vi "acquisition test fixed exposure 5.vi"() -> ()   [LabVIEW 2023]
uses:
  <vilib>/vision/driver/IMAQdx.llb/IMAQdx Attribute Type.ctl
  <vilib>/userDefined/High Color/IMAQdx.ctl
  <vilib>/vision/driver/IMAQdx.llb/IMAQdx Acquisition Mode.ctl
  <vilib>/vision/Avi.llb/IMAQ AVI2 Refnum.ctl
  <vilib>/vision/Image Controls.llb/IMAQ Image.ctl
  <vilib>/vision/driver/IMAQdx.llb/IMAQdx Buffer Number Mode.ctl
  <extravilib>/ChannelInstances/Tag-bool/Read With Abort.vi
  <vilib>/Utility/High Resolution Relative Seconds.vi
  <extravilib>/ChannelInstances/Tag-bool/Write With Abort.vi
  <extravilib>/ChannelInstances/Tag-bool/Instantiate.vi
  <extravilib>/ChannelInstances/Tag-bool/EndpointRead.vi
  <vilib>/vision/EDVR.llb/IMAQ ImageToEDVR.vi
  <vilib>/vision/EDVR.llb/IMAQ ImageToEDVR 1D U8.vi
  <vilib>/vision/EDVR.llb/IMAQ ImageToEDVR 1D I16.vi
  <vilib>/vision/EDVR.llb/IMAQ ImageToEDVR 1D U32.vi
  <vilib>/vision/EDVR.llb/IMAQ ImageToEDVR 1D U16.vi
  <extravilib>/ChannelInstances/Tag-bool/Endpoint.vi
  <vilib>/DAQmx/miscellaneous.llb/DAQmx Fill In Error Info.vi
  <vilib>/DAQmx/configure/timing.llb/DAQmx Timing (Sample Clock).vi
  <vilib>/DAQmx/create/channels.llb/DAQmx Create Channel (AI-Voltage-Basic).vi
  <vilib>/DAQmx/read.llb/DAQmx Read (Analog 1D Wfm NChan NSamp).vi
  <extravilib>/ChannelInstances/Tag-bool.lvlib
  <vilib>/vision/driver/NI_Vision_Acquisition_Software.lvlib
  <resource>/objmgr/imaqdx.rc
panel:
  in  "File Type":enum16{"AVI", "TDMS"}(ring)
  in  "OK Button":bool
  in  "Ring":u16(ring) items=["No TDMS  Codec"]
  out "error out":errorcluster
  in  "Image Type":u16(ring) items=["Grayscale (U8)"=0, "Grayscale (I16)"=1, "Grayscale (U16)"=7, "RGB Color (U32)"=4]
  out "Image 2":T1(plugin-control)
  in  "Buffer Images":i32=30
  out "Optimizations":T2
  in  "Images per File":i64=10000
  out "Images Behind 2":u32
  out "Write Speed":dbl(graph) caption="Image File Write Speed"
  out "Images Acquired Per Second":dbl
  out "Images Saved Per Second":dbl
  out "Maximum FrameRate":dbl
  out "Attribute \nInformation":T4
  out "Sensor Readout Time":dbl
  out "Waveform Chart":waveform(dbl)[](graph)
  in  "stop collection":bool
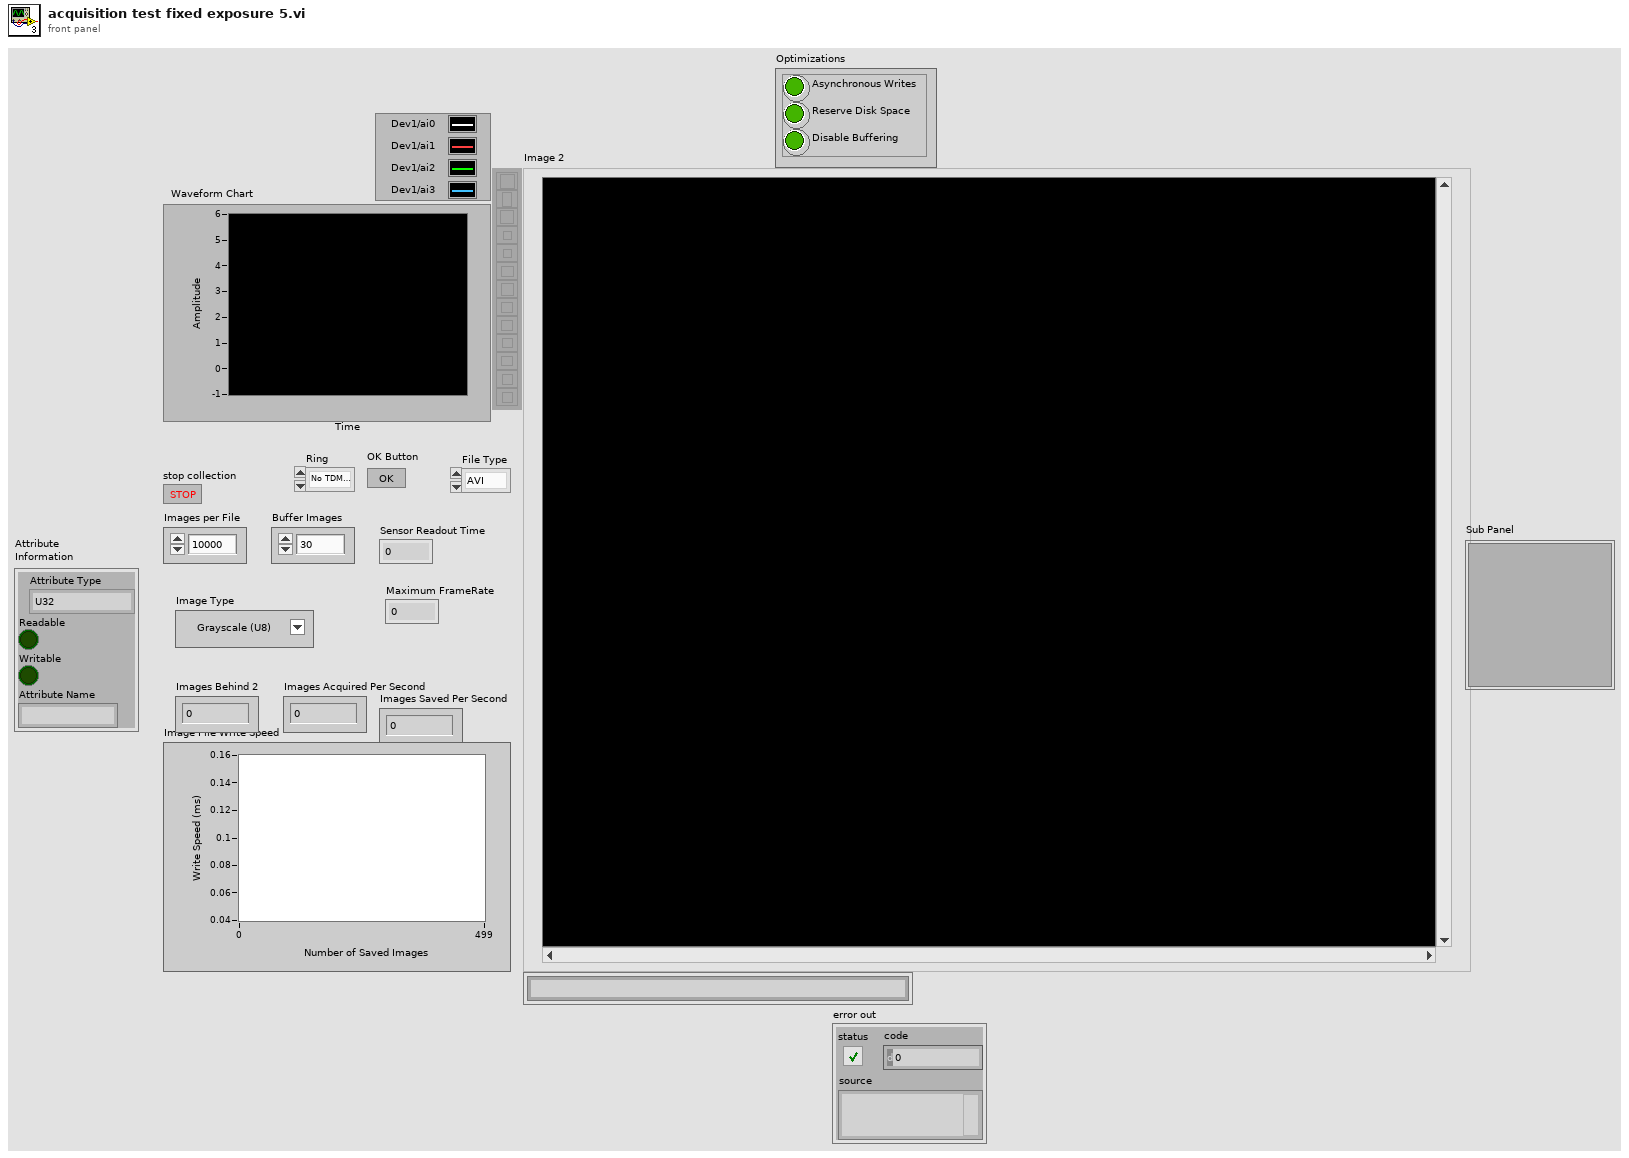
[diagram p1: front panel]
types:
  T1 = typedef "IMAQ Image.ctl" = refnum<image>
  T2 = cluster{"Asynchronous Writes":bool, "Reserve Disk Space":bool, "Disable Buffering":bool}
  T3 = typedef "NI_Vision_Acquisition_Software.lvlib/IMAQdx Attribute Type.ctl" = enum32{"U32", "I64", "DBL", "String", "Enum", "Bool", "Command"}
  T4 = cluster{"Attribute Type":T3, "Readable":bool, "Writable":bool, "Attribute Name":string}
  T5 = typedef "Image Type" = u32
  T6 = typedef "IMAQ AVI2 Refnum.ctl" = refnum<k20>
  T7 = cluster{"Refnum out":refnum<k34>, "Write Settings Out":cluster{"Image Type":T5, "Async File Format":bool}, "AVI Refnum":T6}
  T8 = typedef "NI_Vision_Acquisition_Software.lvlib/IMAQdx Acquisition Mode.ctl" = enum32{"One Shot", "Continuous"}
  T9 = enum16{"Exposure End", "Exposure Center", "Exposure Start", "Start", "NoSync"}
  T10 = typedef "IMAQdx.ctl" = refnum<k21>
  T11 = cluster{"Attribute Type":T3, "Readable":bool, "Writable":bool, "Attribute Name":string}[]
  T12 = cluster{"Image Type":T5, "Async File Format":bool}
  T13 = typedef "Tag-bool.lvlib/))Channel.ctl" = refnum<queue>
  T14 = typedef "NI_Vision_Acquisition_Software.lvlib/IMAQdx Buffer Number Mode.ctl" = enum32{"Next", "Last", "Buffer Number", "Every", "Last New"}
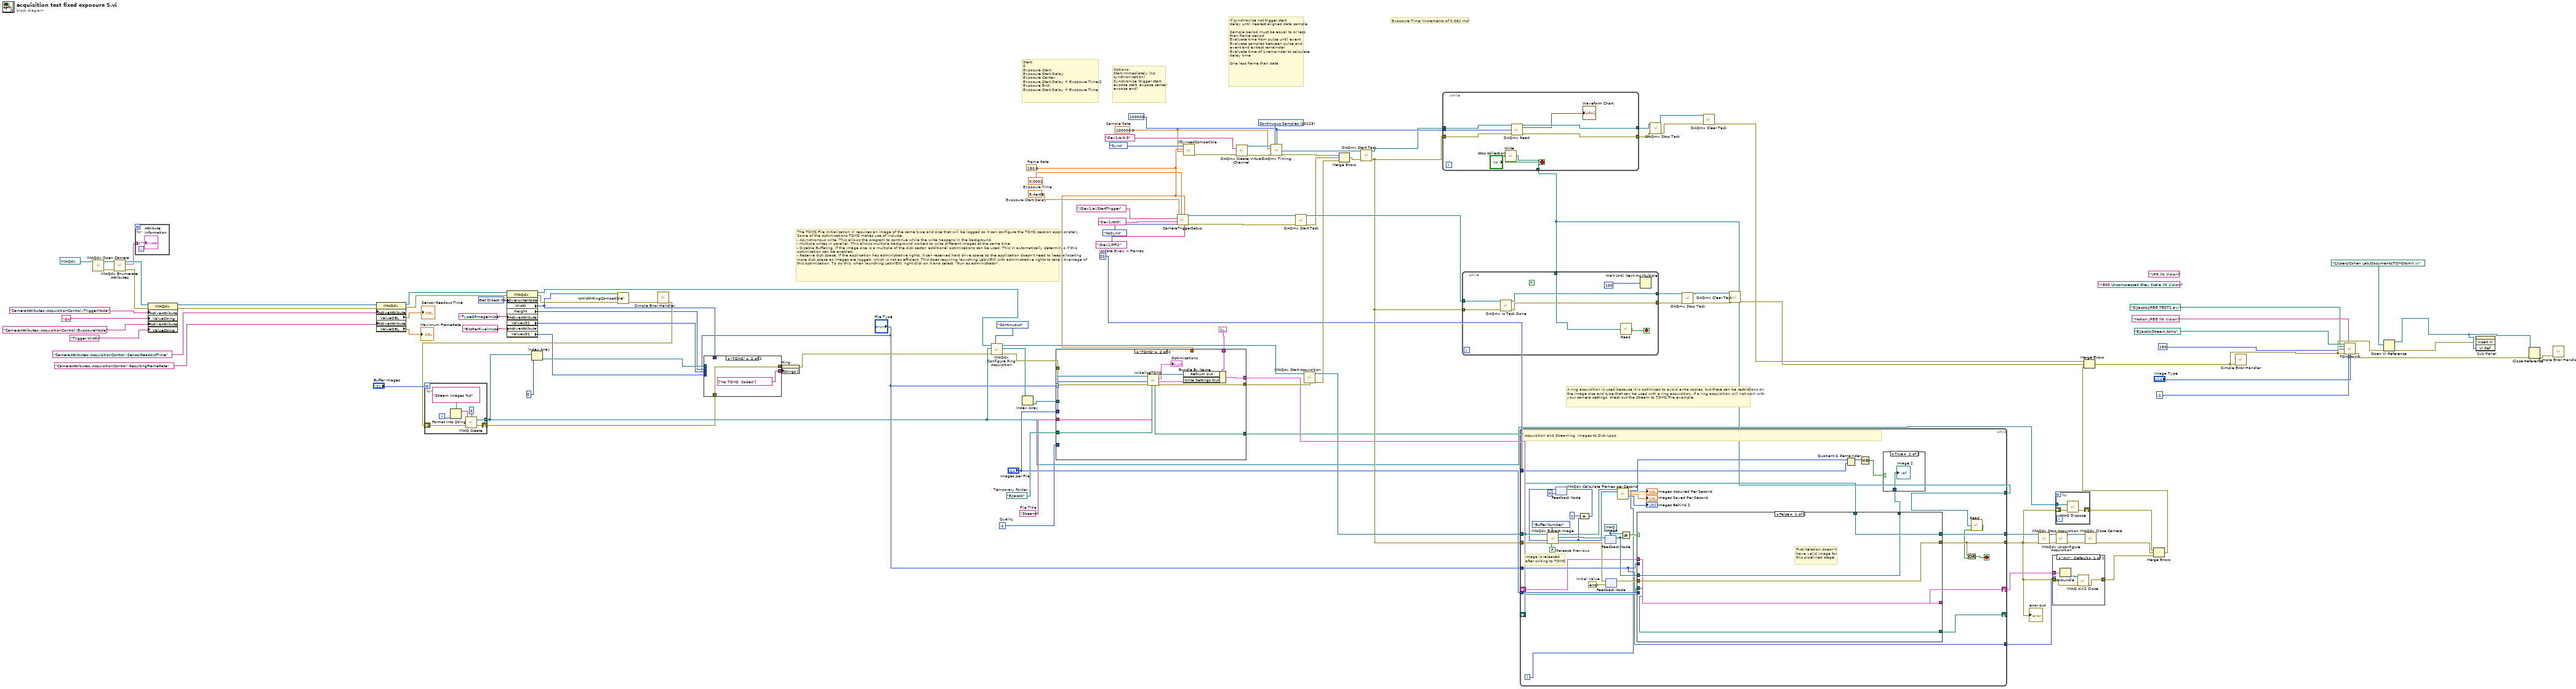
[diagram p0: block diagram]
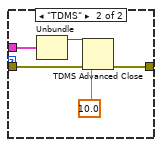
[diagram p2: hidden frame]
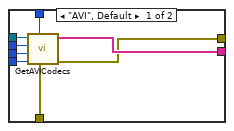
[diagram p3: hidden frame]
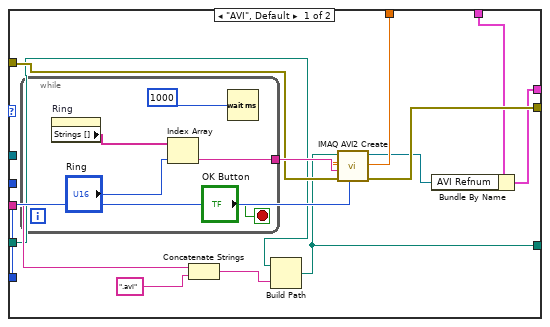
[diagram p4: hidden frame]
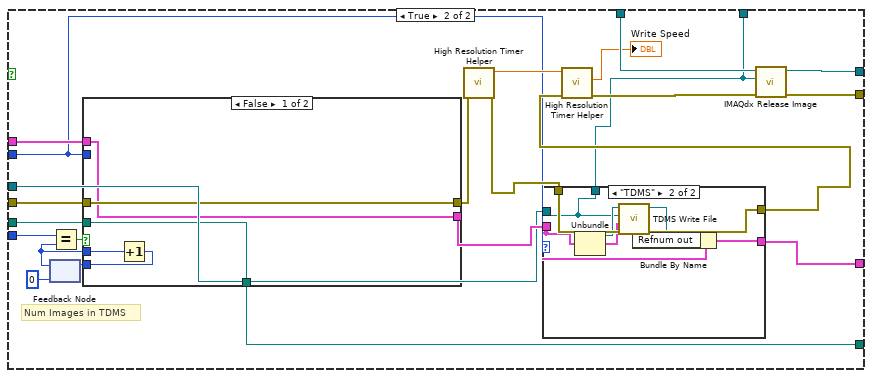
[diagram p6: hidden frame]
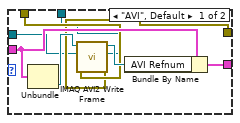
[diagram p7: hidden frame]
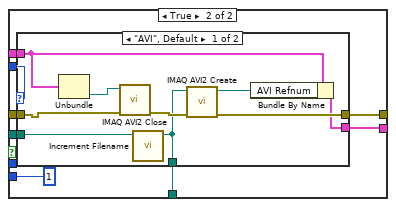
[diagram p8: hidden frame]
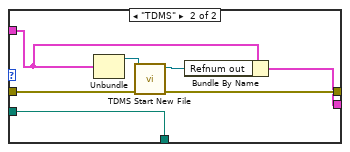
[diagram p9: hidden frame]
diagram:
  w8 = -1  # Quality
  w26 = 20  # Update Every n Frames
  w33 = path "E:/Jacob"  # Temporary Folder
  (unwired) "Y800 Uncompressed Grey Scale (NI Vision)" ("Codec")
  (unwired) "VP9 (NI Vision)" ("Codec")
  w54 = u32 0 items=["Get Oldest"=0, "Fail"=2, "Get Newest"=3] ("OverwriteMode")
  w27 = "Stream"  # File Title
  w82 = 8.4e-06  # Exposure Start Delay
  w1 = 150.0  # Frame Rate
  w81 = 0.0001  # Exposure Time
  w109 = 10123 items=["Finite Samples"=10178, "Continuous Samples"=10123, "Hardware Timed Single Point"=12522] ("sample mode")
  w110 = 100000 ("number of samples per channel")
  w79 = 100000.0  # Sample Rate
  # "The TDMS File Initialization VI requires an image of the same type and size that will be logged so it can configure the TDMS session appropriately. Some of the optimizations TDMS makes use of include:\n- Asynchronous write. This allows the program to continue while the write happens in the background.\n- Multiple writes in parallel. This allows multiple background workers to write different images at the same time.\n- Disable Buffering. If the image size is a multiple of the disk sector, additional optimizations can be used. This VI automatically determines if this optimization can be enabled.\n- Reserve disk space. If the application has administrative rights, it can reserved hard drive space so the application doesn't need to keep allocating more disk space as images are logged, which is not as efficient. This does requiring launching LabVIEW with administrative rights to take advantage of this optimization. To do this, when launching LabVIEW, right click on it and select, \"Run as administrator\"."
  # "A ring acquisition is used because it is optimized to avoid extra copies, but there can be restrictions on the image size and type that can be used with a ring acquisition. If a ring acquisition will not work with your camera settings, check out the Stream to TDMS File example."
  # "Start:\n0\nExposure Start:\nExposure Start Delay\nExposure Center:\nExposure Start Delay + Exposure Time/2\nExposure End:\nExposure Start Delay + Exposure Time"
  # "If synchronize not trigger start\ndelay until nearest aligned data sample\n\nSample period must be equal to or less than frame period\nEvaluate time from pulse until event\nEvaluate samples between pulse and event and extract remainder\nEvaluate time of 1-remainder to calculate delay time\n\nOne less frame than data"
  # "Options:\nStart Immediately (no synchronization)\nSynchronize (trigger start, expose start, expose center, expose end)"
  # "Exposure Time (Increments of 0.061 ms)"
  n1 = call <vilib>:"IMAQdx Open Camera.vi"("Session In"=T10 "cam0") -> ("error out"=w100:errorcluster, "Session Out"=w105:T10)  [unwired: 9 in]
  n2 = call <vilib>:"IMAQdx Enumerate Attributes.vi"("error in"=w100, "Session In"=w105) -> ("error out"=w104:errorcluster, "Attribute Information Array"=w95:T11, "Session Out"=w103:T10)  [unwired: 7 in]
  n3 = for {
    tunnel: w95 -> [w114] mode=indexing
    "Attribute \nInformation" <- w114
  }
  n4 = property class="IMAQdx"(reference=w103, error in=w104, "ActiveAttribute"="CameraAttributes::AcquisitionControl::TriggerMode", "ValueString"="On", "ActiveAttribute"="CameraAttributes::AcquisitionControl::ExposureMode", "ValueString"="Trigger Width") -> (reference out=w97:T10, error out=w96:errorcluster)
  n5 = property class="IMAQdx"(reference=w97, error in=w96, "ActiveAttribute"="CameraAttributes::AcquisitionControl::SensorReadoutTime", "ActiveAttribute"="CameraAttributes::AcquisitionControl::ResultingFrameRate") -> (reference out=w53:T10, error out=w52:errorcluster, "ValueDBL"=→"Sensor Readout Time":dbl, "ValueDBL"=→"Maximum FrameRate":dbl)
  n6 = property class="IMAQdx"(reference=w53, error in=w52, "OverwriteMode"=w54, "ActiveAttribute"="TypeOfImageInUse", "ActiveAttribute"="BitsPerPixelInUse") -> (reference out=w48:T10, error out=w17:errorcluster, "Width"=w21:u32, "Height"=w10:u32, "ValueU32"=w18:u32, "ValueU32"=w19:u32)
  n7 = call "IsWidthRingCompatible.vi"("error in (no error)"=w17, "Width"=w21) -> ("error out"=w13:errorcluster)  [unwired: 9 in]
  n8 = call <vilib>:"Simple Error Handler.vi"("error in (no error)"=w13) -> ("error out"=w12:errorcluster)  [unwired: 4 in, 4 out]
  n9 = for {
    N: "Buffer Images" -> [_]
    tunnel: [w120] -> w23 mode=indexing
    shift-right: [w119] -> w20
    shift-left: w12 -> [w121]
    i -> [w118]
    n10 = Format Into String(format string="Stream Images %d" ("Image Name"), w118) -> (resulting string=w117:string)  [unwired: 2 in, 1 out]
    n11 = call "IMAQ Create"("Border Size"=0, "Image Name"=w117, "error in (no error)"=w121) -> ("New Image"=w120:T1, "error out"=w119:errorcluster)  [unwired: 1 in, 1 out]
  }
  n12 = Index Array(array=w23, index=0) -> (element=w11:T1)
  n13 = case shown="\"TDMS\"" "File Type" {
    tunnel: w21 -> [w129 _]
    tunnel: w20 -> [w128 w131]
    tunnel: w19 -> [w127 _]
    tunnel: w18 -> [w126 _]
    tunnel: [w125 string[] ["No TDMS  Codec"]] -> w16
    tunnel: [w124 w131] -> w15
    tunnel: w11 -> [w123 _]
    tunnel: w10 -> [w122 _]
    frame "AVI", Default {
      n14 = call "GetAVICodecs.vi"("error in (no error)"=w128, "Width"=w129, "Bit Depth"=w127, "Format"=w126, "Height"=w122, "Refnum in"=w123) -> ("error out"=w124:errorcluster, "Codec Names"=w125:string[])  [unwired: 4 in]
    }
    frame "TDMS" {
    }
  }
  n15 = property on="Ring" class="Ring (strict)"(error in=w15, "Strings []"=w16) -> (error out=w14:errorcluster)  [unwired: 1 in, 1 out]
  n16 = call <vilib>:"IMAQdx Configure Ring Acquisition.vi"("Mode"=IMAQdx_Acquisition_Mode."Continuous" ("Continuous?"), "error in"=w14, "Images"=w23, "Session In"=w48) -> ("error out"=w34:errorcluster, "Images Out"=w57:T1[], "Session Out"=w62:T10)  [unwired: 5 in]
  n17 = Index Array(array=w57) -> (element=w56:T1)  [unwired: 1 in]
  n18 = case shown="\"TDMS\"" "File Type" {
    tunnel: "Images per File" -> [_ w161]
    tunnel: w56 -> [_ w160]
    tunnel: [w141 w159] -> w55
    tunnel: w34 -> [w142 w158]
    tunnel: w33 -> [w136 w157]
    tunnel: w27 -> [w138 w156]
    tunnel: w8 -> [w143 _]
    tunnel: w1 -> [w140 _]
    tunnel: [w134 w152] -> w6
    tunnel: T7 {"Refnum out"=refnum, "Write Settings Out"={"Image Type"=0, "Async File Format"=FALSE}, "AVI Refnum"=refnum} ("input cluster") -> [w133 w151]
    tunnel: [w132 w150] -> w3
    frame "AVI", Default {
      n19 = while {
        tunnel: [w147] -> w144
        stop <- "OK Button" stop-if-true
        n20 = property on="Ring" class="Ring (strict)"() -> ("Strings []"=w145:string[])  [unwired: 2 in, 2 out]
        n21 = Index Array(array=w145, index="Ring") -> (element=w147:string)
        n22 = Wait (ms)(milliseconds to wait=u32 1000) -> ()  [unwired: 1 out]
      }
      n23 = Concatenate Strings(w138, ".avi" ("string")) -> (w137:string)
      n24 = Build Path(base path=w136, name or relative path=w137) -> (appended path=w132:path)
      n25 = call "IMAQ AVI2 Create"("Quality"=w143, "error in (no error)"=w142, "Codec"=w144, "Frames Per Second"=w140, "AVI Path"=w132) -> ("error out"=w141:errorcluster, "AVI Refnum"=w135:T6)  [unwired: 5 in]
      n26 = Bundle By Name(cluster=w133, "AVI Refnum"=w135) -> (w134:T7)
    }
    frame "TDMS" {
      n27 = call "InitializeTDMS.vi"("name or relative path"=w156, "Destination Folder"=w157, "error in (no error)"=w158, "Images per File"=w161, "Image Ref in"=w160) -> ("error out"=w159:errorcluster, "Write Settings Out"=w154:T12, "Optimizations"=→"Optimizations":T2, "Refnum out"=w153:refnum<k34>, "appended path"=w150:path)  [unwired: 2 in]
      n28 = Bundle By Name(cluster=w151, "Refnum out"=w153, "Write Settings Out"=w154) -> (w152:T7)
    }
  }
  n29 = call "CameraTriggerSetup.vi"("Camera\nTrigger\nOutput"=tag "/Dev1/PFI2" ("CO.Pulse.Term"), "Frame Rate"=w1, "Sync Type"=T9."NoSync", "Exposure Time"=w81, "Camera\nClock\nCounter"=tag "Dev1/ctr0" ("counter"), "Start Trigger Source"=tag "/Dev1/ai/StartTrigger" ("source"), "Exposure Start Delay"=w82) -> ("error out"=w77:errorcluster, "Refnum out"=w78:refnum<k21>)  [unwired: 3 in]
  n30 = call "IfSyncedCompatible.vi"("Sample Rate"=w79, "Frame Rate"=w1, "Enum"=enum16{"NoSync", "Sync"}."Sync") -> ("error out"=w2:errorcluster)  [unwired: 8 in]
  n31 = call-poly <vilib>:"DAQmx Create Virtual Channel.vi"("physical channels"=tag "Dev1/ai0:3", "error in"=w2) -> ("task out"=w113:refnum<k21>, "error out"=w112:errorcluster)  [unwired: 12 in]
  n32 = call-poly <vilib>:"DAQmx Timing.vi"("task/channels in"=w113, "sample mode"=w109, "samples per channel"=w110, "rate"=w79, "error in"=w112) -> ("task out"=w75:refnum<k21>, "error out"=w73:errorcluster)  [unwired: 9 in]
  n33 = call <vilib>:"DAQmx Start Task.vi"("task/channels in"=w78, "error in"=w77) -> ("task out"=w76:refnum<k21>, "error out"=w71:errorcluster)  [unwired: 12 in]
  n34 = call <vilib>:"IMAQdx Start Acquisition.vi"("error in"=w55, "Session In"=w62) -> ("error out"=w50:errorcluster, "Session Out"=w59:T10)  [unwired: 8 out]
  n35 = Merge Errors(w73, w71, w50) -> (w72:errorcluster)
  n36 = call <vilib>:"DAQmx Start Task.vi"("task/channels in"=w75, "error in"=w72) -> ("task out"=w74:refnum<k21>, "error out"=w49:errorcluster)  [unwired: 12 in]
  n37 = while {
    tunnel: [w169] -> w93
    tunnel: [w168] -> w92
    tunnel: w74 -> [w167]
    tunnel: w49 -> [w166]
    tunnel: w110 -> [w165]
    tunnel: [w162] -> w47
    stop <- "stop collection" stop-if-true
    n38 = call <extravilib>:"Write.vi"("element"="stop collection") -> ("channel"=w162:T13)  [unwired: 1 out]
    n39 = call-poly <vilib>:"DAQmx Read.vi"("task/channels in"=w167, "number of samples per channel"=w165, "error in"=w166) -> ("task out"=w169:refnum<k21>, "data"=→"Waveform Chart":waveform(dbl)[], "error out"=w168:errorcluster)  [unwired: 10 in]
  }
  n40 = while {
    tunnel: w47 -> [w170]
    tunnel: w76 -> [w175]
    tunnel: w49 -> [w174]
    tunnel: [w173] -> w89
    tunnel: [w172] -> w88
    stop <- w176 stop-if-true
    (unwired) TRUE ("auto start")
    n41 = call <vilib>:"DAQmx Is Task Done.vi"("task/channels in"=w175, "error in"=w174) -> ("task out"=w173:refnum<k21>, "error out"=w172:errorcluster)  [unwired: 11 in, 1 out]
    n42 = call <extravilib>:"Read.vi"("channel"=w170) -> ("element"=w176:bool)  [unwired: 1 in, 1 out]
    n43 = Wait Until Next ms Multiple(millisecond multiple=u32 100) -> ()  [unwired: 1 out]
  }
  n44 = while {
    tunnel: w49 -> [w212]
    tunnel: w59 -> [w210]
    tunnel: [w211] -> w60
    tunnel: [w199] -> w39
    tunnel: "Images per File" -> [w197]
    tunnel: w47 -> [w184]
    tunnel: "File Type" -> [w179]
    tunnel: w26 -> [w182]
    shift-right: [w180] -> w4
    shift-left: w6 -> [w181]
    tunnel: [w179] -> w5
    shift-right: [w177] -> _
    shift-left: w3 -> [w178]
    i -> [w186]
    stop <- w201 stop-if-true
    w189 = errorcluster {"status"=FALSE, "code"=0, "source"=""}  # Initial Value
    w208 = FALSE  # Release Previous
    w204 = T1 refnum ("Image Out")
    # "Image is released after writing to TDMS."
    # "Acquisition and Streaming  Images to Disk Loop"
    n45 = feedback #1(u32 0) -> (w191:u32)
    n46 = call <vilib>:"IMAQdx Extract Image.vi"("Release Previous (true)"=w208, "Buffer Number Mode (Next)"=IMAQdx_Buffer_Number_Mode."Buffer Number" ("Buffer Number Mode"), "error in"=w212, "Buffer Number In"=w191, "Session In"=w210) -> ("error out"=w198:errorcluster, "Buffer Number Out"=w193:u32, "Image Out"=w206:T1, "Session Out"=w207:T10)  [unwired: 3 in]
    n47 = Compound Arithmetic op=ADD(u32 1 ("value"), w193) -> (w194:u32)
    n48 = feedback-in #1(w194) -> ()
    n49 = feedback-in #2(w206) -> ()
    n50 = feedback #2(w204) -> (w202:T1)
    n51 = feedback-in #3(w198) -> ()
    n52 = feedback #3(w189) -> (w205:errorcluster)
    n53 = call <vilib>:"IMAQdx Calculate Frames per Second.vi"("Session In"=w207, "Buffer Number"=w193) -> ("Acquired Frames per Second"=→"Images Acquired Per Second":dbl, "Processed Frames per Second"=→"Images Saved Per Second":dbl, "Images Behind"=→"Images Behind 2":i32)  [unwired: 7 in, 4 out]
    n54 = Not Equal?(x=w204, y=w202) -> (x != y?=w203:bool)
    n55 = case shown="False" w203 {
      tunnel: w202 -> [w216 w222]
      tunnel: w205 -> [w217 w237]
      tunnel: [w218 w241] -> w211
      tunnel: w210 -> [w218 w240]
      tunnel: [w217 w239] -> w199
      tunnel: w197 -> [_ w235]
      tunnel: [w216 w223] -> w185
      tunnel: w179 -> [_ w221]
      tunnel: w181 -> [w215 w228]
      tunnel: [w215 w227] -> w180
      tunnel: w178 -> [w214 w220]
      tunnel: [w214 w219] -> w177
      frame False {
        # "First iteration doesn't have valid image for this pipelined stage."
      }
      frame True {
        # "Num Images in TDMS"
        n56 = feedback #4(i64 0) -> (w234:i64)
        n57 = Equal?(x=w235, y=w234) -> (x = y?=w236:bool)
        n58 = case shown="False" w236 {
          tunnel: [w262 i64 1] -> w233
          tunnel: w237 -> [w261 w268]
          tunnel: [w261 w269] -> w232
          tunnel: w234 -> [w260 _]
          tunnel: w221 -> [_ w267]
          tunnel: w228 -> [w259 w266]
          tunnel: [w259 w265] -> w226
          tunnel: w220 -> [w258 w264]
          tunnel: [w258 w263] -> w219
          frame False {
            n59 = Increment(x=w260) -> (x+1=w262:i64)
          }
          frame True {
            n60 = case shown="\"AVI\", Default" w267 {
              tunnel: [w277 w286] -> w269
              tunnel: w268 -> [w278 w285]
              tunnel: w266 -> [w273 w281]
              tunnel: [w276 w282] -> w265
              tunnel: w264 -> [w272 w280]
              tunnel: [w271 w280] -> w263
              frame "AVI", Default {
                n61 = Unbundle(w273) -> ("AVI Refnum"=w275:T6)  [unwired: 2 out]
                n62 = call "IMAQ AVI2 Close"("error in (no error)"=w278, "AVI Refnum"=w275) -> ("error out"=w279:errorcluster)  [unwired: 9 in]
                n63 = call "Increment Filename.vi"("Path In"=w272) -> ("Incremented Path Out"=w271:path)  [unwired: 10 in]
                n64 = call "IMAQ AVI2 Create"("error in (no error)"=w279, "AVI Path"=w271) -> ("error out"=w277:errorcluster, "AVI Refnum"=w274:T6)  [unwired: 8 in]
                n65 = Bundle By Name(cluster=w273, "AVI Refnum"=w274) -> (w276:T7)
              }
              frame "TDMS" {
                n66 = Unbundle(w281) -> ("Refnum out"=w284:refnum<k34>)  [unwired: 2 out]
                n67 = call "TDMS Start New File.vi"("error in"=w285, "Previous TDMS Refnum In"=w284) -> ("error out"=w286:errorcluster, "New TDMS Refnum Out"=w283:refnum<k34>)  [unwired: 8 in]
                n68 = Bundle By Name(cluster=w281, "Refnum out"=w283) -> (w282:T7)
              }
            }
          }
        }
        n69 = feedback-in #4(w233) -> ()
        n70 = call "High Resolution Timer Helper.vi"("error in (no error)"=w232) -> ("error out"=w225:errorcluster, "Current Time"=w231:dbl)  [unwired: 8 in, 1 out]
        n71 = case shown="\"TDMS\"" w221 {
          tunnel: w225 -> [w246 w257]
          tunnel: [w245 w256] -> w224
          tunnel: w222 -> [w243 w250]
          tunnel: w226 -> [w247 w253]
          tunnel: [w244 w251] -> w227
          tunnel: [w242 w250] -> w223
          frame "AVI", Default {
            n72 = Unbundle(w247) -> ("AVI Refnum"=w249:T6)  [unwired: 2 out]
            n73 = call "IMAQ AVI2 Write Frame"("error in (no error)"=w246, "Image"=w243, "AVI Refnum"=w249) -> ("error out"=w245:errorcluster, "Image Out (duplicate)"=w242:T1, "AVI Refnum (duplicate)"=w248:T6)  [unwired: 6 in]
            n74 = Bundle By Name(cluster=w247, "AVI Refnum"=w248) -> (w244:T7)
          }
          frame "TDMS" {
            n75 = Unbundle(w253) -> ("Refnum out"=w255:refnum<k34>, "Write Settings Out"=w254:T12)  [unwired: 1 out]
            n76 = call "TDMS Write File.vi"("error in"=w257, "Write Settings"=w254, "Image"=w250, "TDMS Ref In"=w255) -> ("error out"=w256:errorcluster, "TDMS Ref Out"=w252:refnum<k34>)  [unwired: 6 in]
            n77 = Bundle By Name(cluster=w253, "Refnum out"=w252) -> (w251:T7)
          }
        }
        n78 = call "High Resolution Timer Helper.vi"("error in (no error)"=w224, "Previous Time"=w231) -> ("error out"=w230:errorcluster, "Time Difference (ms)"=→"Write Speed":dbl)  [unwired: 7 in, 1 out]
        n79 = call <vilib>:"IMAQdx Release Image.vi"("error in"=w230, "Image"=w223, "Session In"=w240) -> ("error out"=w239:errorcluster, "Session Out"=w241:T10)  [unwired: 7 in]
      }
    }
    n80 = Quotient & Remainder(x=w186, y=w182) -> (x-y*floor(x/y)=w188:i32)  [unwired: 1 out]
    n81 = Equal To 0?(x=w188) -> (x = 0?=w187:bool)
    n82 = case shown="True" w187 {
      tunnel: w185 -> [_ w213]
      frame False {
      }
      frame True {
        "Image 2" <- w213
      }
    }
    n83 = call <extravilib>:"Read.vi"("channel"=w184) -> ("element"=w183:bool)  [unwired: 1 in, 1 out]
    n84 = Or(x=w199, y=w183) -> (x .or. y?=w201:bool)
  }
  "error out" <- w39
  n85 = call <vilib>:"DAQmx Stop Task.vi"("task/channels in"=w93, "error in"=w92) -> ("task out"=w91:refnum<k21>, "error out"=w70:errorcluster)  [unwired: 12 in]
  n86 = call <vilib>:"DAQmx Stop Task.vi"("task/channels in"=w89, "error in"=w88) -> ("task out"=w94:refnum<k21>, "error out"=w69:errorcluster)  [unwired: 12 in]
  n87 = call <vilib>:"DAQmx Clear Task.vi"("task in"=w91, "error in"=w70) -> ("error out"=w68:errorcluster)  [unwired: 13 in]
  n88 = call <vilib>:"DAQmx Clear Task.vi"("task in"=w94, "error in"=w69) -> ("error out"=w67:errorcluster)  [unwired: 13 in]
  n89 = call <vilib>:"IMAQdx Stop Acquisition.vi"("error in"=w39, "Session In"=w60) -> ("error out"=w63:errorcluster, "Session Out"=w64:T10)  [unwired: 8 out]
  n90 = case shown="\"AVI\", Default" w5 {
    tunnel: [w287 w294] -> w42
    tunnel: w39 -> [w288 w293]
    tunnel: w4 -> [w290 w292]
    frame "AVI", Default {
      n91 = Unbundle(w290) -> ("AVI Refnum"=w289:T6)  [unwired: 2 out]
      n92 = call "IMAQ AVI2 Close"("error in (no error)"=w288, "AVI Refnum"=w289) -> ("error out"=w287:errorcluster)  [unwired: 9 in]
    }
    frame "TDMS" {
      n93 = Unbundle(w292) -> ("Refnum out"=w291:refnum<k34>)  [unwired: 2 out]
      n94 = TDMS Advanced Close(6:10.0 ("timeout (10 s)"), 8:w293, 11:w291) -> (0:w294:errorcluster)  [unwired: 1 in, 1 out]
    }
  }
  n95 = for {
    shift-right: [w297] -> w40
    shift-left: w39 -> [w298]
    tunnel: w23 -> [w296] mode=indexing
    n96 = call "IMAQ Dispose"("Image"=w296, "error in (no error)"=w298) -> ("error out"=w297:errorcluster)  [unwired: 4 in]
  }
  n97 = call <vilib>:"IMAQdx Unconfigure Acquisition.vi"("error in"=w63, "Session In"=w64) -> ("error out"=w66:errorcluster, "Session Out"=w65:T10)  [unwired: 8 out]
  n98 = call <vilib>:"IMAQdx Close Camera.vi"("error in"=w66, "Session In"=w65) -> ("error out"=w41:errorcluster)  [unwired: 9 out]
  n99 = Merge Errors(w40, w41, w42) -> (w32:errorcluster)
  n100 = Merge Errors(w68, w67, w32) -> (w37:errorcluster)
  n101 = call <vilib>:"Simple Error Handler.vi"("error in (no error)"=w37) -> ()  [unwired: 4 in, 5 out]
  n102 = call "TDMStoAVI.vi"("TDMS Path"=path "E:/Jacob/Stream.tdms" ("AVI Path"), "Codec"="Motion JPEG (NI Vision)", "AVI Out Path"=path "D:/Jacob/JPEG TEST2.avi" ("AVI Path"), "Frames Per Second"=u32 150, "error in (no error)"=w37, "Quality"=-1, "Image Type"="Image Type") -> ("error out"=w36:errorcluster)  [unwired: 8 in]
  n103 = Open VI Reference(vi path=path "C:/Users/Cohen Lab/Documents/TDMStoAVI.vi", error in (no error)=w37) -> (vi reference=w43:refnum<vi>, error out=w38:errorcluster)  [unwired: 4 in]
  n104 = invoke on="Sub Panel" class="SubPnl" method="Insert VI"(error in=w38, "VI Ref"=w43) -> ()  [unwired: 2 in, 4 out]
  n105 = Close Reference(reference=w43, error in (no error)=w36) -> (error out=w35:errorcluster)
  n106 = call <vilib>:"Simple Error Handler.vi"("error in (no error)"=w35) -> ()  [unwired: 4 in, 5 out]
